vi "freq_measure_diag.vi"(10 "Ref_average":dbl, 11 "data":dbl[](array[numeric])) -> (1 "Actual (last) Rising edge index":i32, 2 "First Rising edge index":i32, 3 "Rising edges":i32)   [LabVIEW 2013]
panel:
  out "Waveform Graph":dbl[](graph)
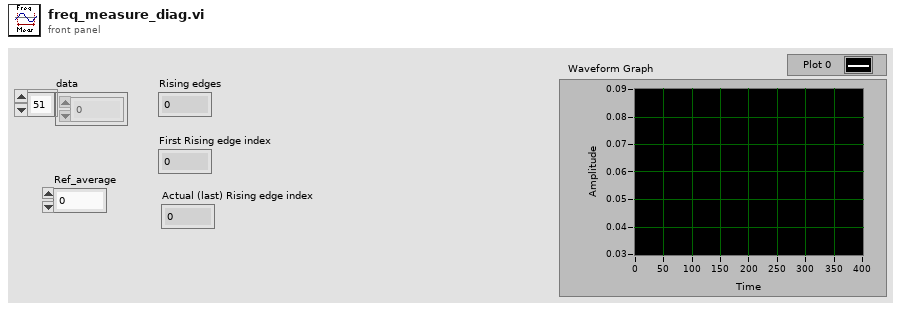
[diagram p1: front panel]
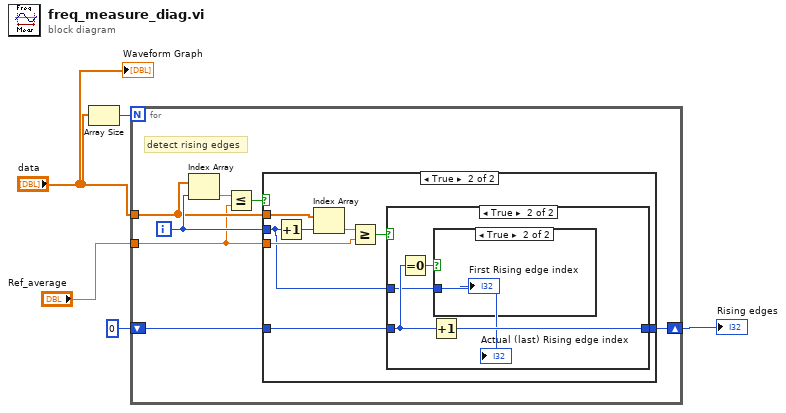
[diagram p0: block diagram]
diagram:
  n1 = Array Size(array="data") -> (size(s)=w3:i32)
  n2 = for {
    N: w3 -> [_]
    tunnel: "data" -> [w10]
    shift-right: [w8] -> w5
    shift-left: 0 -> [w9]
    tunnel: "Ref_average" -> [w6]
    i -> [w11]
    # "detect rising edges"
    n3 = Index Array(array=w10, index=w11) -> (element=w7:dbl)
    n4 = Less Or Equal?(x=w7, y=w6) -> (x <= y?=w12:bool)
    n5 = case shown="True" w12 {
      tunnel: w11 -> [_ w14]
      tunnel: w10 -> [_ w21]
      tunnel: w9 -> [w13 w18]
      tunnel: [w13 w17] -> w8
      tunnel: w6 -> [_ w15]
      frame False {
      }
      frame True {
        n6 = Increment(x=w14) -> (x+1=w20:i32)
        n7 = Index Array(array=w21, index=w20) -> (element=w16:dbl)
        n8 = Greater Or Equal?(x=w16, y=w15) -> (x >= y?=w19:bool)
        n9 = case shown="True" w19 {
          tunnel: w18 -> [w22 w25]
          tunnel: [w22 w26] -> w17
          tunnel: w14 -> [_ w23]
          frame False {
          }
          frame True {
            n10 = Equal To 0?(x=w25) -> (x = 0?=w24:bool)
            n11 = Increment(x=w25) -> (x+1=w26:i32)
            n12 = case shown="True" w24 {
              tunnel: w23 -> [_ w27]
              frame False {
              }
              frame True {
                "First Rising edge index" <- w27
              }
            }
            "Actual (last) Rising edge index" <- w23
          }
        }
      }
    }
  }
  "Rising edges" <- w5
  "Waveform Graph" <- "data"
